vi "New__slk_mt.vi"(8 "error in (no error)":errorcluster, 11 "case model in":refnum<class "CaseModel__slk_mt.lvclass">) -> (0 "error out":errorcluster, 3 "adapter out":refnum<class "DatatypeAdapter__slk_mt.lvclass">)   [LabVIEW 2012, in "Lazyboots Menu Tool.lvlib" / "DatatypeAdapter__slk_mt.lvclass"]
doc: "Creates a new adapter object by specified case model object."
uses:
  DatatypeAdapter__slk_mt.lvclass
  CaseModel/CaseModel__slk_mt.lvclass
  BooleanAdapter/BooleanAdapter__slk_mt.lvclass
  NumericAdapter/NumericAdapter__slk_mt.lvclass
  StringAdapter/StringAdapter__slk_mt.lvclass
panel:
  # "New__slk_mt.vi\nCreates a new adapter object by specified case model object.\n\nNOTICE -- YOU MUST LEAVE THIS NOTICE IN PLACE.\n\nCopyright (c) 2011, LIANG LIU Shawn.Liu.cn@gmail.com\nAll rights reserved.\n\nRedistribution and use in source and binary forms, with or without modification, are permitted provided that the following conditions are met:\n-Redistributions of source code must retain the above copyright notice, this list of conditions and the following disclaimer.\n-Redistributions in binary form must reproduce the above copyright notice, this list of conditions and the following disclaimer in the documentation and/or other materials provided with the distribution.\n-Neither the name of the eLp nor the names of its contributors may be used to endorse or promote products derived from this software without specific prior written permission.\n\nTHIS SOFTWARE IS PROVIDED BY THE COPYRIGHT HOLDERS AND CONTRIBUTORS \"AS IS\" AND ANY EXPRESS OR IMPLIED WARRANTIES, INCLUDING, BUT NOT LIMITED TO, THE IMPLIED WARRANTIES OF MERCHANTABILITY AND FITNESS FOR A PARTICULAR PURPOSE ARE DISCLAIMED. IN NO EVENT SHALL THE COPYRIGHT HOLDER OR CONTRIBUTORS BE LIABLE FOR ANY DIRECT, INDIRECT, INCIDENTAL, SPECIAL, EXEMPLARY, OR CONSEQUENTIAL DAMAGES (INCLUDING, BUT NOT LIMITED TO, PROCUREMENT OF SUBSTITUTE GOODS OR SERVICES; LOSS OF USE, DATA, OR PROFITS; OR BUSINESS INTERRUPTION) HOWEVER CAUSED AND ON ANY THEORY OF LIABILITY, WHETHER IN CONTRACT, STRICT LIABILITY, OR TORT (INCLUDING NEGLIGENCE OR OTHERWISE) ARISING IN ANY WAY OUT OF THE USE OF THIS SOFTWARE, EVEN IF ADVISED OF THE POSSIBILITY OF SUCH DAMAGE."
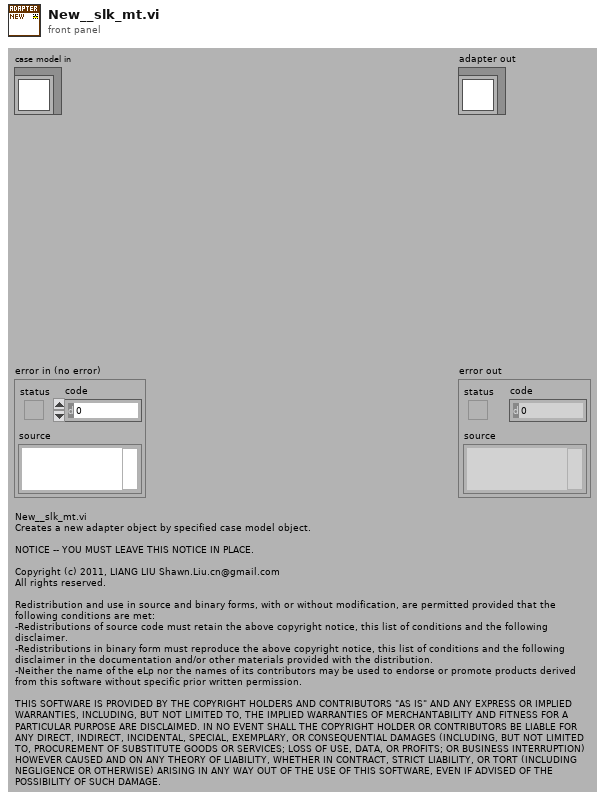
[diagram p1: front panel]
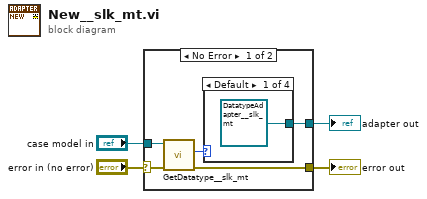
[diagram p0: block diagram]
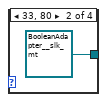
[diagram p2: hidden frame]
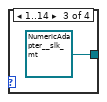
[diagram p3: hidden frame]
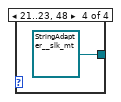
[diagram p4: hidden frame]
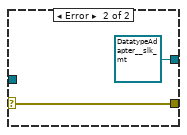
[diagram p5: hidden frame]
diagram:
  n1 = case shown="No Error" "error in (no error)" {
    selector: "error in (no error)" -> [w9 w15]
    tunnel: [w8 w15] -> w3
    tunnel: [w7 refnum<class "DatatypeAdapter__slk_mt.lvclass"> refnum ("CaseMonitor.lvlib:DatatypeAdapter.lvclass")] -> w2
    tunnel: "case model in" -> [w6 _]
    frame No Error {
      n2 = call "GetDatatype__slk_mt.vi"("error in (no error)"=w9, "case model in"=w6) -> ("error out"=w8:errorcluster, "data type"=w5:u8)  [unwired: 7 in, 1 out]
      n3 = case shown="Default" w5 {
        tunnel: [refnum<class "DatatypeAdapter__slk_mt.lvclass"> refnum ("CaseMonitor.lvlib:DatatypeAdapter.lvclass") refnum<class "BooleanAdapter__slk_mt.lvclass"> refnum ("CaseMonitor.lvlib:BooleanAdapter.lvclass") refnum<class "NumericAdapter__slk_mt.lvclass"> refnum ("CaseMonitor.lvlib:NumericAdapter.lvclass") refnum<class "StringAdapter__slk_mt.lvclass"> refnum ("CaseMonitor.lvlib:StringAdapter.lvclass")] -> w7
        frame Default {
        }
        frame 33, 80 {
        }
        frame 1..14 {
        }
        frame 21..23, 48 {
        }
      }
    }
    frame Error {
    }
  }
  "error out" <- w3
  "adapter out" <- w2
